vi "VisionCode.vi"(0 "Image Src":T1=refnum, 1 "error in (no error)":errorcluster) -> (2 "Image Out":T1(plugin-control), 3 "error out":errorcluster, 4 "Particle Measurements (Pixels)":dbl[][](array[numeric])=[[375.7939059158945, 403.03617248752676, 200.0, 0.0]] format="%.2f")   [LabVIEW 2012]
uses:
  <vilib>/vision/Image Controls.llb/IMAQ Image.ctl
  <vilib>/vision/NI_Vision_Development_Module.lvlib
panel:
  in  "Blue":cluster{"Lower":i32, "Upper":i32}={"Lower"=93, "Upper"=255} {"Upper" scale=0.0..255.0; "Lower" scale=0.0..255.0}
  in  "Red":cluster{"Lower":i32, "Upper":i32}={"Lower"=0, "Upper"=217} {"Upper" scale=0.0..255.0; "Lower" scale=0.0..255.0}
  in  "Green":cluster{"Lower":i32, "Upper":i32}={"Lower"=155, "Upper"=255} {"Upper" scale=0.0..255.0; "Lower" scale=0.0..255.0}
  out "Heights":sgl[](array[numeric])
  out "numOfTargets":i32=1
  out "Target Heights":cluster{"X":sgl, "Y":sgl}[][](array[cluster])
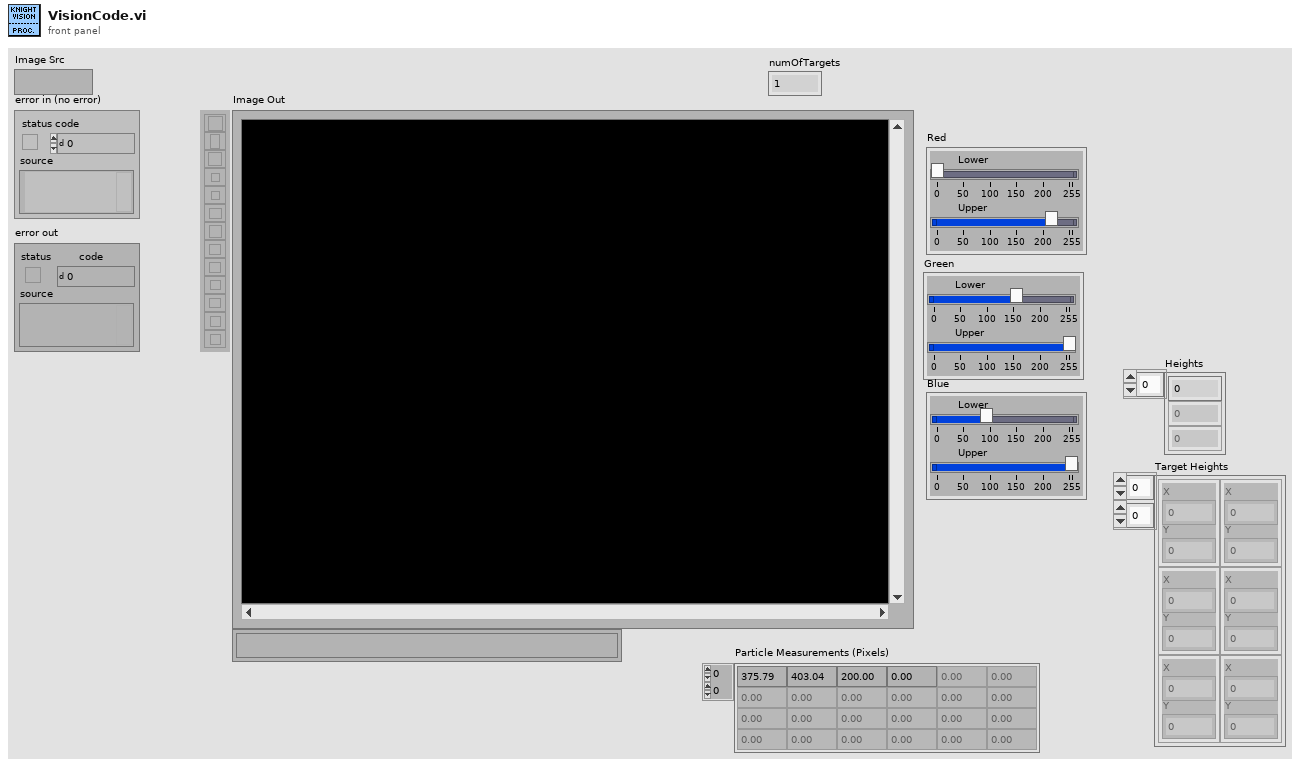
[diagram p1: front panel]
types:
  T1 = typedef "IMAQ Image.ctl" = refnum<image>
  T2 = typedef "Particle Parameters" = i32
  T3 = cluster{"Measurement Parameter":i32, "Range Lower Value":dbl, "Range Upper Value":dbl, "Range":bool, "Measurement Type":bool}[]
  T4 = enum16{"Get First Edge", "Get First + Last Edge", "Get All Edges"}
  T5 = cluster{"Level Type":enum32{"Absolute Value", "Relative value"}, "Threshold Level":i32, "Hysteresis":i32}
  T6 = cluster{"ID":enum32{"External", "Internal"}, "Type":u32, i32[]}
  T7 = cluster{"ID":enum32{"External", "Internal"}, "Type":u32, i32[]}[]
  T8 = cluster{i32[], cluster{"ID":enum32{"External", "Internal"}, "Type":u32, i32[]}[]}
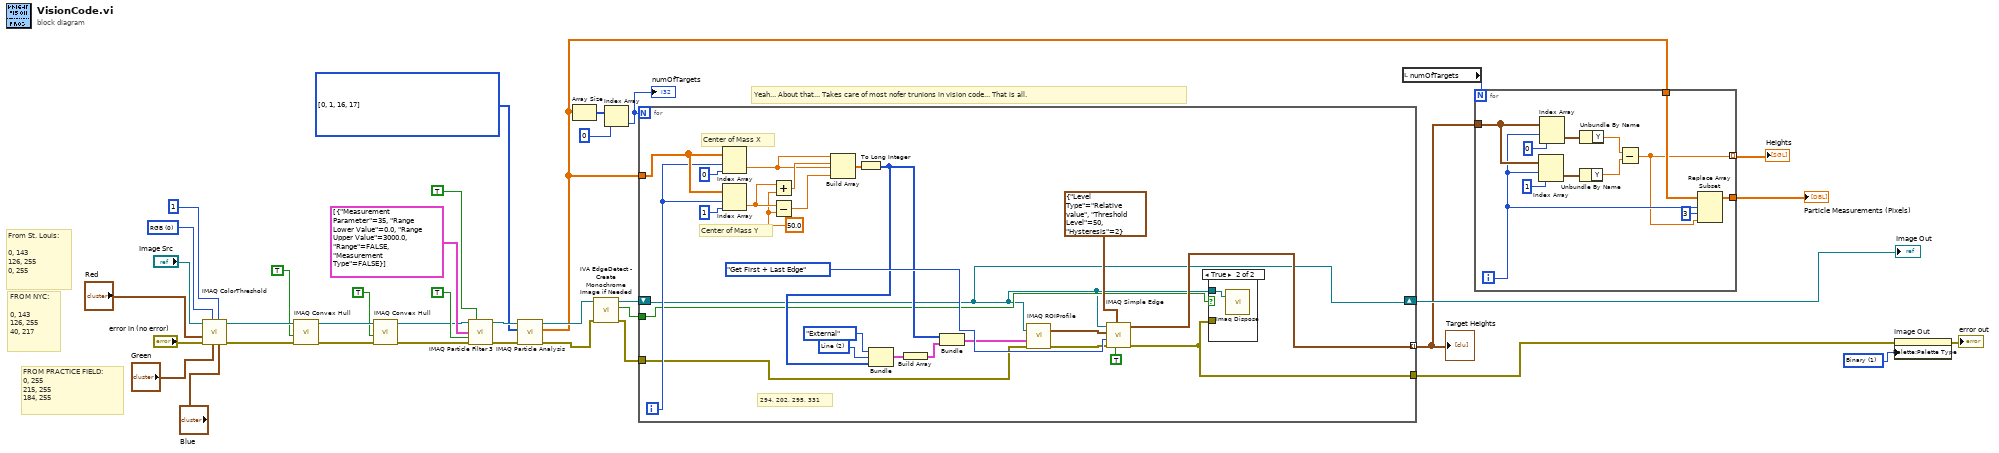
[diagram p0: block diagram]
diagram:
  w16 = T2[] [0, 1, 16, 17] items=["Center of Mass X", "Center of Mass Y", "First Pixel X", "First Pixel Y", "Bounding Rect Left", "Bounding Rect Top", "Bounding Rect Right", "Bounding Rect Bottom", "Max Feret Diameter Start X", "Max Feret Diameter Start Y", "Max Feret Diameter End X", "Max Feret Diameter End Y", "Max Horiz. Segment Length Left", "Max Horiz. Segment Length Right", "Max Horiz. Segment Length Row", "-", "Bounding Rect Width", "Bounding Rect Height", "Bounding Rect Diagonal", "Perimeter", "Convex Hull Perimeter", "Holes' Perimeter", "Max Feret Diameter", "Equivalent Ellipse Major Axis", "Equivalent Ellipse Minor Axis", "Equivalent Ellipse Minor Axis (Feret)", "Equivalent Rect Long Side", "Equivalent Rect Short Side", "Equivalent Rect Diagonal", "Equivalent Rect Short Side (Feret)", "Average Horiz. Segment Length", "Average Vert. Segment Length", "Hydraulic Radius", "Waddel Disk Diameter", "-", "Area", "Holes' Area", "Particle & Holes' Area", "Convex Hull Area", "Image Area", "-", "Number of Holes", "Number of Horiz. Segments", "Number of Vert. Segments", "-", "Orientation", "Max Feret Diameter Orientation", "-", "% Area/Image Area", "% Area/(Particle & Holes' Area)", "Ratio of Equivalent Ellipse Axes", "Ratio of Equivalent Rect Sides", "-", "Elongation Factor", "Compactness Factor", "Heywood Circularity Factor", "Type Factor", "-", "Sum X", "Sum Y", "Sum XX", "Sum XY", "Sum YY", "Sum XXX", "Sum XXY", "Sum XYY", "Sum YYY", "-", "Moment of Inertia XX", "Moment of Inertia XY", "Moment of Inertia YY", "Moment of Inertia XXX", "Moment of Inertia XXY", "Moment of Inertia XYY", "Moment of Inertia YYY", "Norm. Moment of Inertia XX", "Norm. Moment of Inertia XY", "Norm. Moment of Inertia YY", "Norm. Moment of Inertia XXX", "Norm. Moment of Inertia XXY", "Norm. Moment of Inertia XYY", "Norm. Moment of Inertia YYY", "Hu Moment 1", "Hu Moment 2", "Hu Moment 3", "Hu Moment 4", "Hu Moment 5", "Hu Moment 6", "Hu Moment 7"] ("Pixel Measurements")
  w31 = u32 1 items=["Grayscale", "Binary", "Gradient", "Rainbow", "Temperature", "User Defined"] ("Palette")
  w37 = u16 0 items=["RGB", "HSL", "HSV", "HSI"] ("Color Mode")
  # "FROM NYC:\n\n0, 143\n126, 255\n40, 217"
  # "FROM PRACTICE FIELD:\n0, 255\n215, 255\n184, 255"
  # "From St. Louis:\n\n0, 143\n126, 255\n0, 255"
  # "Yeah... About that... Takes care of most nofer trunions in vision code... That is all."
  n1 = call "IMAQ ColorThreshold"("Blue or Luma or Val or Inten Range"="Blue", "Replace Value"=1, "Green or Sat Range"="Green", "Color Mode"=w37, "error in (no error)"="error in (no error)", "Red or Hue Range"="Red", "Image Src"="Image Src") -> ("error out"=w33:errorcluster, "Image Dst Out"=w32:T1)  [unwired: 1 in, 2 out]
  n2 = call "IMAQ Convex Hull"("error in (no error)"=w33, "Connectivity 4/8 (8)"=TRUE, "Image Src"=w32) -> ("error out"=w27:errorcluster, "Image Dst Out"=w26:T1)  [unwired: 1 in, 6 out]
  n3 = call "IMAQ Convex Hull"("error in (no error)"=w27, "Connectivity 4/8 (8)"=TRUE, "Image Src"=w26) -> ("error out"=w21:errorcluster, "Image Dst Out"=w20:T1)  [unwired: 1 in, 6 out]
  n4 = call "IMAQ Particle Filter 3"("Image Src"=w20, "Connectivity 4/8 (8)"=TRUE, "Selection Values"=T3 [{"Measurement Parameter"=35, "Range Lower Value"=0.0, "Range Upper Value"=3000.0, "Range"=FALSE, "Measurement Type"=FALSE}], "Keep/Remove Particles (F)"=TRUE ("Keep/Remove Particles"), "error in (no error)"=w21) -> ("Image Dst Out"=w18:T1, "error out"=w17:errorcluster)  [unwired: 4 in, 5 out]
  n5 = call "IMAQ Particle Analysis"("error in (no error)"=w17, "Pixel Measurements"=w16, "Image"=w18) -> ("error out"=w13:errorcluster, "Particle Measurements (Pixels)"=w2:dbl[][], "Image Out (duplicate)"=w14:T1)  [unwired: 3 in, 3 out]
  n6 = Array Size(array=w2) -> (size(s)=w11:i32[])
  n7 = call <vilib>:"IVA EdgeDetect - Create Monochrome Image if Needed.vi"("error in (no error)"=w13, "Image In"=w14) -> ("error out"=w7:errorcluster, "Mono Image Created"=w8:bool, "Mono Image Out"=w9:T1)  [unwired: 7 out]
  n8 = Index Array(array=w11, index=0) -> (element=w5:i32)
  "numOfTargets" <- w5
  n9 = for {
    N: w5 -> [_]
    tunnel: w7 -> [w41]
    tunnel: w2 -> [w58]
    tunnel: [w43] -> w6 mode=indexing
    shift-right: [w40] -> w15
    shift-left: w9 -> [w40]
    tunnel: w8 -> [w42]
    tunnel: [w39] -> w12
    i -> [w57]
    w47 = u32 2 items=["No Selection", "Point", "Line", "Rectangle", "Oval", "Polygon", "Freehand Region", "Annulus", "Unused2", "Unused3", "Broken Line", "Freehand Line", "Rotated Rectangle"] ("Type")
    w53 = 50.0 ("y")
    # "294, 202, 295, 331"
    # "Center of Mass Y"
    # "Center of Mass X"
    n10 = Index Array(array=w58, index (row)=w57, index (col)=0 ("disabled index (col)")) -> (element=w51:dbl)
    n11 = Index Array(array=w58, index (row)=w57, index (col)=1 ("disabled index (col)")) -> (element=w55:dbl)
    n12 = Add(x=w55, y=w53) -> (x+y=w54:dbl)
    n13 = Subtract(x=w55, y=w53) -> (x-y=w52:dbl)
    n14 = Build Array(w51, w54, w51, w52) -> (w50:dbl[])
    n15 = To Long Integer(number=w50) -> (32bit integer=w44:i32[])
    n16 = Bundle("ID"=enum32{"External", "Internal"}."External", "Type"=w47, w44) -> (w46:T6)  [unwired: 1 in]
    n17 = Build Array(w46) -> (w45:T7)
    n18 = Bundle(w44, w45) -> (w49:T8)  [unwired: 1 in]
    n19 = call "IMAQ ROIProfile"("error in (no error)"=w41, "ROI Descriptor"=w49, "Image"=w40) -> ("error out"=w60:errorcluster, "Pixel Coordinates"=w61:cluster{"X":u32, "Y":u32}[])  [unwired: 4 out]
    n20 = call "IMAQ Simple Edge"("Sub-Pixel Accuracy"=TRUE, "Threshold Parameters"=T5 {"Level Type"=enum."Relative value", "Threshold Level"=50, "Hysteresis"=2}, "error in (no error)"=w60, "Process"=T4."Get First + Last Edge", "Pixel Coordinates"=w61, "Image Src"=w40) -> ("error out"=w39:errorcluster, "Edges Coordinates"=w43:cluster{"X":sgl, "Y":sgl}[])  [unwired: 4 out]
    n21 = case shown="True" w42 {
      tunnel: w40 -> [_ w65]
      tunnel: w39 -> [_ _]
      frame False {
      }
      frame True {
        n22 = call "Imaq Dispose"("Image"=w65) -> ()  [unwired: 2 in, 4 out]
      }
    }
  }
  "Image Out" <- w15
  "Target Heights" <- w6
  n23 = local read "numOfTargets"() -> (w4:i32)
  n24 = for {
    N: w4 -> [_]
    tunnel: w6 -> [w73]
    tunnel: [w66] -> w3 mode=indexing
    tunnel: w2 -> [w70]
    tunnel: [w67] -> w1
    i -> [w69]
    n25 = Index Array(array=w73, index (row)=w69, index (col)=1 ("disabled index (col)")) -> (element=w75:cluster{"X":sgl, "Y":sgl})
    n26 = Index Array(array=w73, index (row)=w69, index (col)=0 ("disabled index (col)")) -> (element=w77:cluster{"X":sgl, "Y":sgl})
    n27 = Unbundle By Name(w75) -> ("Y"=w71:sgl)
    n28 = Unbundle By Name(w77) -> ("Y"=w72:sgl)
    n29 = Subtract(x=w72, y=w71) -> (x-y=w66:sgl)
    n30 = Replace Array Subset(array=w70, new element=w66, index (row)=w69, index (col)=3 ("disabled index (col)")) -> (w67:dbl[][])
  }
  "Particle Measurements (Pixels)" <- w1
  "Heights" <- w3
  n31 = property on="Image Out" class="ImageControl"(error in=w12, "Palette:Palette Type"=w31) -> (error out=→"error out":errorcluster)  [unwired: 1 in, 1 out]
